vi "Read Data(IL).vi"(8 "error in (no error)":errorcluster, 9 "timeout (0)":dbl=20.0 format="%.2g", 10 "number to read (-1)":i32=3, 11 "LIN Device in":T1={"Master Frame(3C)"="MasterReq\nSPA3414_ConfigurationsCMAGeely_CEMCALYPSOSDB34XX0Cfg_LIN3_190709_", "Slave Frame(3D)"="SlaveResp\nSPA3414_ConfigurationsCMAGeely_CEMCALYPSOSDB34XX0Cfg_LIN3_190709_", "Request Schedule"="CEMLIN3DiagRequestSchedule\nSPA3414_ConfigurationsCMAGeely_CEMCALYPSOSDB34XX0Cfg_LIN3_190709_", "Response Schedule"="CEMLIN3DiagResponseSchedule\nSPA3414_ConfigurationsCMAGeely_CEMCALYPSOSDB34XX0Cfg_LIN3_190709_", "Frame Write SCU"="", "Frame Read SCU"="", "LIN Name"=""}) -> (0 "error out":errorcluster, 1 "LIN comm":T2 {"communication state" items=["Idle", "Active", "Inactive"]; "fault code" format="%08x"; "last error" items=["None", "Unknown ID", "Form", "Framing", "Readback", "Timeout", "Checksum"]}, 2 "data":T5[](array[typedef]) {"event ID" format="%x"; "payload" format="%x"; "timestamp" format="%<%.7X\n%x>T"; "type" items=["LIN Data"=64, "LIN Bus Error"=65, "LIN No Response"=66, "Delay"=224, "Log Trigger"=225, "Start Trigger"=226]; "identifier" format="%x"}, 3 "LIN Device out":T1={"Master Frame(3C)"="MasterReq\nSPA3414_ConfigurationsCMAGeely_CEMCALYPSOSDB34XX0Cfg_LIN3_190709_", "Slave Frame(3D)"="SlaveResp\nSPA3414_ConfigurationsCMAGeely_CEMCALYPSOSDB34XX0Cfg_LIN3_190709_", "Request Schedule"="CEMLIN3DiagRequestSchedule\nSPA3414_ConfigurationsCMAGeely_CEMCALYPSOSDB34XX0Cfg_LIN3_190709_", "Response Schedule"="CEMLIN3DiagResponseSchedule\nSPA3414_ConfigurationsCMAGeely_CEMCALYPSOSDB34XX0Cfg_LIN3_190709_", "Frame Write SCU"="", "Frame Read SCU"="", "LIN Name"=""})   [LabVIEW 2018]
uses:
  <vilib>/xnet/xnet.llb/XNET Frame LIN.ctl
  <vilib>/xnet/xnet.llb/XNET Frame Type LIN.ctl
  <vilib>/xnet/xnet.llb/XNET LIN Comm.ctl
  <vilib>/xnet/xnet.llb/XNET LIN Comm State.ctl
  <vilib>/xnet/xnet.llb/XNET LIN Last Err.ctl
  LIN Device.ctl
  <vilib>/xnet/xnet.llb/XNET Write (State LIN Schedule Change).vi
  <vilib>/xnet/xnet.llb/XNET Read (State LIN Comm).vi
  <vilib>/xnet/xnet.llb/XNET Read (Frame LIN).vi
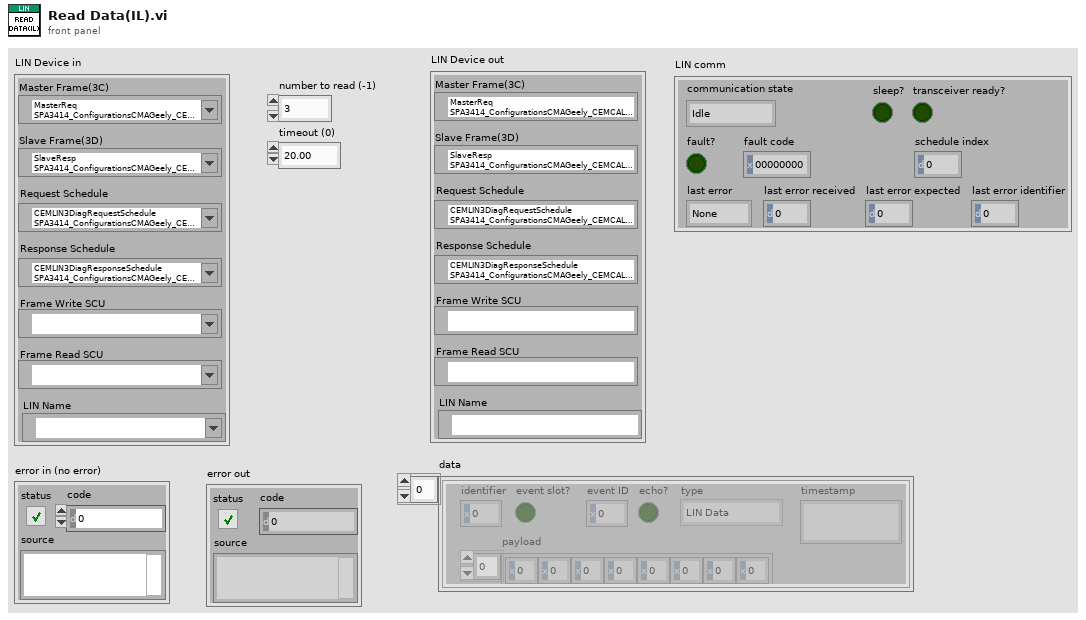
[diagram p1: front panel]
types:
  T1 = typedef "LIN Device.ctl" = cluster{"Master Frame(3C)":refnum<k21>, "Slave Frame(3D)":refnum<k21>, "Request Schedule":refnum<k21>, "Response Schedule":refnum<k21>, "Frame Write SCU":refnum<k21>, "Frame Read SCU":refnum<k21>, "LIN Name":refnum<k21>}
  T2 = typedef "XNET LIN Comm.ctl" = cluster{"fault code":i32, "fault?":bool, "communication state":T3, "last error":T4, "last error received":u8, "last error expected":u8, "last error identifier":u8, "sleep?":bool, "transceiver ready?":bool, "schedule index":u8}
  T3 = typedef "XNET LIN Comm State.ctl" = u8
  T4 = typedef "XNET LIN Last Err.ctl" = u8
  T5 = typedef "XNET Frame LIN.ctl" = cluster{"timestamp":timestamp, "payload":u8[], "identifier":u32, "type":T6, "event ID":u8, "event slot?":bool, "echo?":bool}
  T6 = typedef "XNET Frame Type LIN.ctl" = u8
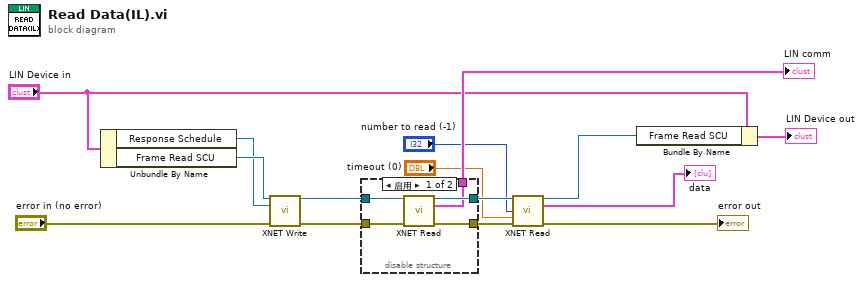
[diagram p0: block diagram]
diagram:
  n1 = Unbundle By Name("LIN Device in") -> ("Response Schedule"=w4:refnum<k21>, "Frame Read SCU"=w5:refnum<k21>)
  n2 = call-poly <vilib>:"XNET Write.vi"("session in"=w5, "data"=w4, "error in (no error)"="error in (no error)") -> ("session out"=w13:refnum<k21>, "error out"=w14:errorcluster)  [unwired: 11 in]
  n3 = disable-structure shown="启用" {
    disable-tunnel: w14 -> [w20 w21]
    disable-tunnel: w13 -> [w19 w22]
    disable-tunnel: [w18 w22] -> w12
    disable-tunnel: [w17 w21] -> w11
    disable-tunnel: [w16 _] -> w10
    frame Enabled {
      n4 = call-poly <vilib>:"XNET Read.vi"("session in"=w19, "error in (no error)"=w20) -> ("session out"=w18:refnum<k21>, "LIN comm"=w16:T2, "error out"=w17:errorcluster)  [unwired: 11 in]
    }
    frame Disabled {
    }
  }
  "LIN comm" <- w10
  n5 = call-poly <vilib>:"XNET Read.vi"("session in"=w12, "number to read (-1)"="number to read (-1)", "timeout (0)"="timeout (0)", "error in (no error)"=w11) -> ("session out"=w9:refnum<k21>, "data"=→"data":T5[], "error out"=→"error out":errorcluster)  [unwired: 8 in, 1 out]
  n6 = Bundle By Name(cluster="LIN Device in", "Frame Read SCU"=w9) -> (→"LIN Device out":T1)
